vi "udp_mutlicast_test.vi"() -> ()   [LabVIEW 2010]
uses:
  <vilib>/Utility/tcp.llb/UDP Multicast Open.vi
panel:
  in  "button:stop":bool
  in  "button:send":bool
  in  "Send to Port":u16=58432
  in  "Multicast Address":string="234.5.6.7"
  in  "data":string="Hello World!"
  in  "TTL":u16=1
  in  "Local Port":u16=58431
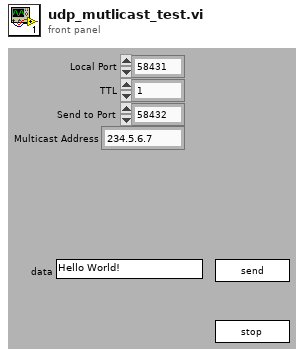
[diagram p1: front panel]
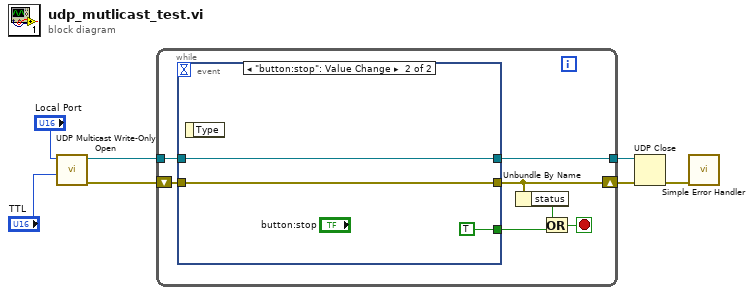
[diagram p0: block diagram]
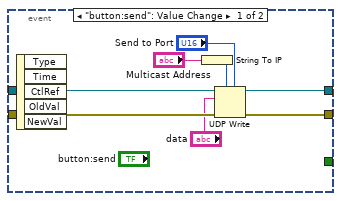
[diagram p2: hidden frame]
diagram:
  n1 = call-poly <vilib>:"UDP Multicast Write-Only Open.vi"("time-to-live (1)"="TTL", "port"="Local Port") -> ("error out"=w5:errorcluster, "connection ID"=w4:refnum<k16>)  [unwired: 8 in]
  n2 = while {
    tunnel: w4 -> [w13]
    tunnel: [w12] -> w2
    shift-right: [w11] -> w3
    shift-left: w5 -> [w14]
    stop <- w8 stop-if-true
    n3 = event shown="[1] \"button:stop\": Value Change" {
      selector: _ -> [_ _]
      dyn-events: _ -> [_ _]
      timeout: _ -> [_ _]
      tunnel: w14 -> [w22 w24]
      tunnel: w13 -> [w21 w25]
      tunnel: [w16 w24] -> w11
      tunnel: [w15 w25] -> w12
      tunnel: [_ TRUE] -> w9
      event "button:send": Value Change {
        n4 = event-data() -> ()  [unwired: 1 in, 5 out]
        n5 = String To IP(1:"Multicast Address") -> (0:w17:u32)
        n6 = UDP Write(address=w17, port or service name="Send to Port", connection ID=w21, data in="data", 8:w22) -> (error out=w16:errorcluster, 3:w15:refnum<k16>)  [unwired: 1 in]
      }
      event "button:stop": Value Change {
        n7 = event-data() -> ()  [unwired: 1 in, 1 out]
      }
    }
    n8 = Unbundle By Name(w11) -> ("status"=w10:bool)
    n9 = Or(x=w10, y=w9) -> (x .or. y?=w8:bool)
  }
  n10 = UDP Close(connection ID=w2, 8:w3) -> (error out=w1:errorcluster)  [unwired: 1 out]
  n11 = call <vilib>:"Simple Error Handler.vi"("error in (no error)"=w1) -> ()  [unwired: 4 in, 5 out]
